vi "UPDATE VI UL NM.vi"(9 "Array":string[](array[string]), 10 "columns":string[](array[string]), 11 "TABELLA":string) -> (3 "String":string)   [LabVIEW 2019]
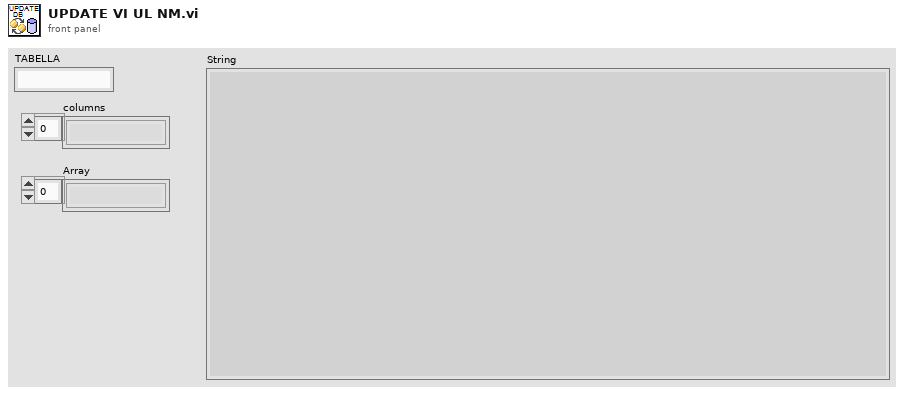
[diagram p1: front panel]
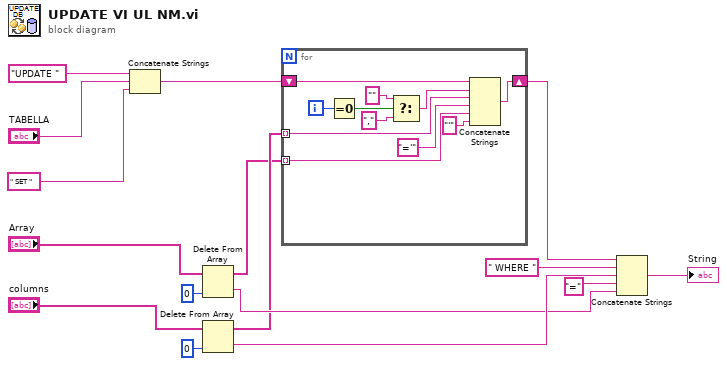
[diagram p0: block diagram]
diagram:
  n1 = Concatenate Strings("UPDATE ", "TABELLA", " SET " ("string")) -> (w16:string)
  n2 = Delete From Array(array="Array", index=0) -> (deleted portion=w4:string, array with subset deleted=w1:string[])  [unwired: 1 in]
  n3 = Delete From Array(array="columns", index=0) -> (deleted portion=w6:string, array with subset deleted=w2:string[])  [unwired: 1 in]
  n4 = for {
    tunnel: w2 -> [w27] mode=indexing
    shift-right: [w20] -> w12
    shift-left: w16 -> [w22]
    tunnel: w1 -> [w18] mode=indexing
    i -> [w26]
    n5 = Equal To 0?(x=w26) -> (x = 0?=w25:bool)
    n6 = Select(t="" ("String"), s=w25, f=",") -> (s? t:f=w21:string)
    n7 = Concatenate Strings(w22, w21, w27, "='" ("string"), w18, "'" ("string")) -> (w20:string)
  }
  n8 = Concatenate Strings(w12, " WHERE " ("string"), w6, "=" ("string"), w4) -> (→"String":string)
